vi "Search Library by UID.vi"(8 "error in (no error)":errorcluster, 10 "UID":string, 11 "SongLibrary":refnum<class "SongLibrary.lvclass">) -> (0 "error out":errorcluster, 1 "Index":i32, 2 "Song":refnum<class "Song.lvclass">, 3 "SongLibraryOut":refnum<class "SongLibrary.lvclass">, 5 "Found?":bool)   [LabVIEW 2015, in "SongLibrary.lvclass"]
uses:
  SongLibrary.lvclass
  Song/Song.lvclass
  MusicElementLibrary.lvclass/MusicElementLibrary.ctl
  MusicElement.lvclass/MusicElement.ctl
  MusicElement.lvclass
  MusicElementLibrary.lvclass
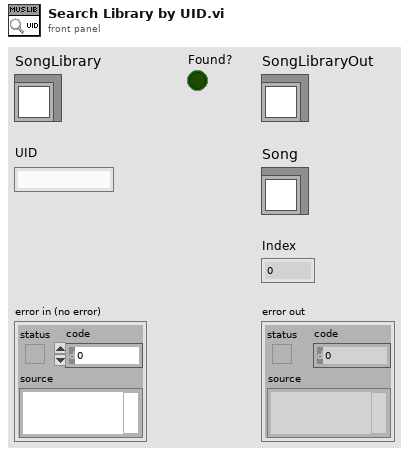
[diagram p1: front panel]
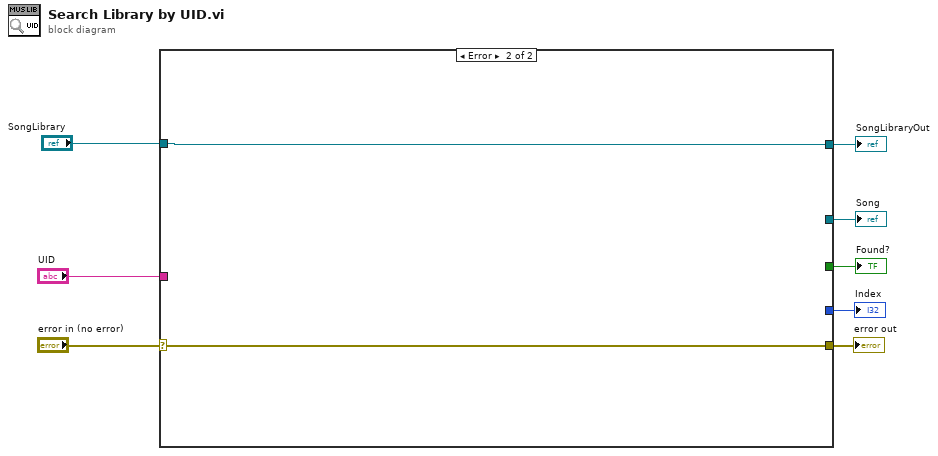
[diagram p0: block diagram]
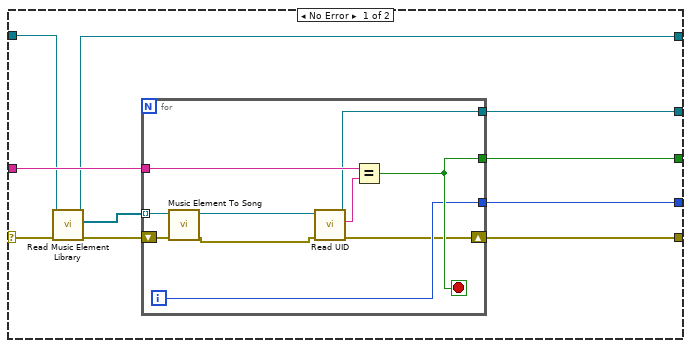
[diagram p2: hidden frame]
diagram:
  n1 = case shown="Error" "error in (no error)" {
    selector: "error in (no error)" -> [w13 w30]
    tunnel: [w18 w30] -> w7
    tunnel: "UID" -> [w17 _]
    tunnel: [w16 _] -> w2
    tunnel: [w15 _] -> w5
    tunnel: [w14 _] -> w4
    tunnel: "SongLibrary" -> [w12 w29]
    tunnel: [w9 w29] -> w1
    frame No Error {
      n2 = call "Read Music Element Library.vi"("error in (no error)"=w13, "MusicElementLibrary in"=w12) -> ("error out"=w11:errorcluster, "Music Element Library"=w10:refnum<class "MusicElement.lvclass">[], "MusicElementLibrary out"=w9:refnum<class "SongLibrary.lvclass">)  [unwired: 7 in]
      n3 = for {
        shift-right: [w25] -> w18
        shift-left: w11 -> [w22]
        tunnel: w17 -> [w28]
        tunnel: [w24] -> w16
        tunnel: [w27] -> w15
        tunnel: [w26] -> w14
        tunnel: w10 -> [w21] mode=indexing
        i -> [w26]
        stop <- w27 stop-if-true
        n4 = call "Music Element To Song.vi"("error in (no error)"=w22, "MusicElement"=w21) -> ("error out"=w19:errorcluster, "Song out"=w20:refnum<class "Song.lvclass">)  [unwired: 8 in]
        n5 = call "Read UID.vi"("error in (no error)"=w19, "MusicElement in"=w20) -> ("error out"=w25:errorcluster, "UID"=w23:string, "MusicElement out"=w24:refnum<class "Song.lvclass">)  [unwired: 7 in]
        n6 = Equal?(x=w28, y=w23) -> (x = y?=w27:bool)
      }
    }
    frame Error {
    }
  }
  "error out" <- w7
  "Found?" <- w5
  "Index" <- w4
  "SongLibraryOut" <- w1
  "Song" <- w2
